vi "PictureCtrlDefault.vi"(1 "picture in":picture) -> (0 "Pause if TRUE":bool)   [LabVIEW 2020]
doc: "Displays the picture."
panel:
  out "Bad picture":T1
  out "picture out":picture
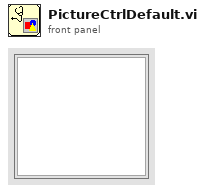
[diagram p1: front panel]
types:
  T1 = cluster{"Picture is empty or invalid":string, "Left:":i16, "Top:":i16, "Right:":i16, "Bottom:":i16}
  T2 = enum16{"Always On", "Always Off", "Off While Running"}
  T3 = typedef "imagedata.ctl" = cluster{"image type":i32, "image depth":i32, "image":u8[], "mask":u8[], "colors":u32[], "Rectangle":cluster{"left":i16, "top":i16, "right":i16, "bottom":i16}}
  T4 = typedef "LVBoundsTypeDef.ctl" = cluster{"Width":u32, "Height":u32}
  T5 = cluster{string, "left":i16, "top":i16, "right":i16, "bottom":i16}
  T6 = typedef "LVRectTypeDef.ctl" = cluster{"Left":i16, "Top":i16, "Right":i16, "Bottom":i16}
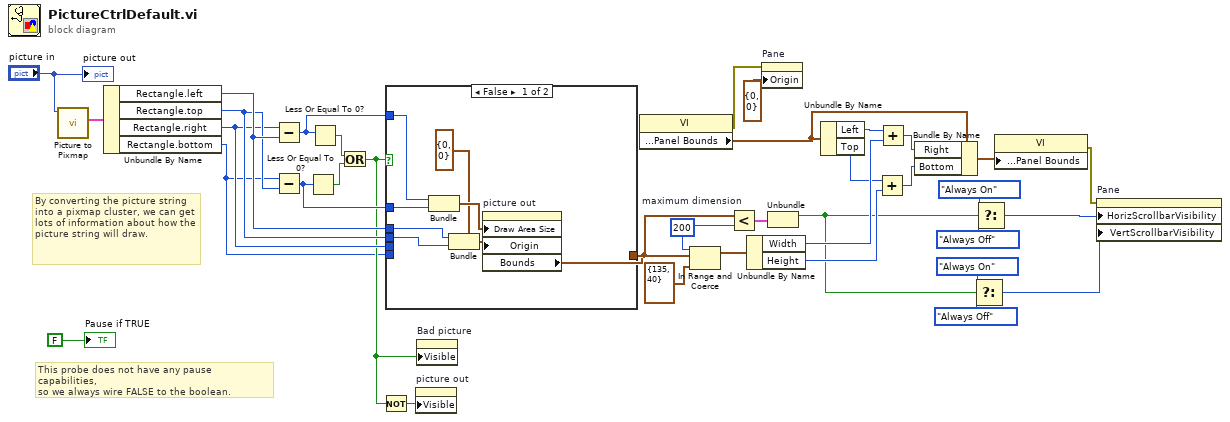
[diagram p0: block diagram]
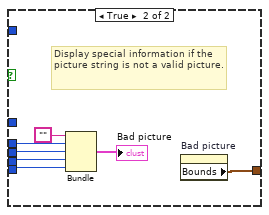
[diagram p2: hidden frame]
diagram:
  w17 = i16 200  # maximum dimension
  # "This probe does not have any pause capabilities,\nso we always wire FALSE to the boolean."
  # "By converting the picture string into a pixmap cluster, we can get lots of information about how the picture string will draw."
  n1 = call <vilib>:"Picture to Pixmap.vi"("picture"="picture in") -> ("image data"=w36:T3)  [unwired: 9 in, 1 out]
  n2 = Unbundle By Name(w36) -> ("Rectangle.left"=w32:i16, "Rectangle.top"=w31:i16, "Rectangle.right"=w30:i16, "Rectangle.bottom"=w13:i16)
  n3 = Subtract(x=w30, y=w32) -> (x-y=w29:i16)
  n4 = Subtract(x=w13, y=w31) -> (x-y=w28:i16)
  n5 = Less Or Equal To 0?(x=w28) -> (x <= 0?=w33:bool)
  n6 = Less Or Equal To 0?(x=w29) -> (x <= 0?=w34:bool)
  n7 = Or(x=w34, y=w33) -> (x .or. y?=w19:bool)
  n8 = Not(x=w19) -> (.not. x?=w18:bool)
  n9 = case shown="False" w19 {
    tunnel: w32 -> [w38 w50]
    tunnel: w31 -> [w37 w49]
    tunnel: w30 -> [_ w48]
    tunnel: w13 -> [_ w47]
    tunnel: [w41 w45] -> w16
    tunnel: w29 -> [w42 _]
    tunnel: w28 -> [w43 _]
    frame False {
      n10 = Bundle(w42, w43) -> (w44:cluster{i16, i16})  [unwired: 1 in]
      n11 = Bundle(cluster=cluster{"Horizontal":i16, "Vertical":i16} {"Horizontal"=0, "Vertical"=0} ("Origin"), "Horizontal"=w38, "Vertical"=w37) -> (w40:cluster{"Horizontal":i16, "Vertical":i16})
      n12 = property on="picture out" class="Pict"("Draw Area Size"=w44, "Origin"=w40) -> ("Bounds"=w41:T4)  [unwired: 2 in, 2 out]
    }
    frame True {
      # "Display special information if the picture string is not a valid picture."
      n13 = Bundle("", "left"=w50, "top"=w49, "right"=w48, "bottom"=w47) -> (→"Bad picture":T5)  [unwired: 1 in]
      n14 = property on="Bad picture" class="Clust (strict)"() -> ("Bounds"=w45:T4)  [unwired: 2 in, 2 out]
    }
  }
  n15 = property on="picture out" class="Pict"("Visible"=w18) -> ()  [unwired: 2 in, 2 out]
  n16 = property on="Bad picture" class="Clust (strict)"("Visible"=w19) -> ()  [unwired: 2 in, 2 out]
  n17 = property class="VI"() -> (error out=w12:errorcluster, "Front Panel Window:Panel Bounds"=w10:T6)  [unwired: 2 in, 1 out]
  n18 = In Range and Coerce(upper limit=w17, x=w16, lower limit=cluster{"Width":u32, "Height":u32} {"Width"=135, "Height"=40}) -> (coerced(x)=w21:T4)  [unwired: 1 out]
  n19 = Less?(x=w16, y=w17) -> (x < y?=w15:cluster{"Width":bool, "Height":bool})
  n20 = Unbundle By Name(w21) -> ("Width"=w26:u32, "Height"=w24:u32)
  n21 = property on="Pane" class="Pane"(error in=w12, "Origin"=cluster{"Horizontal":i16, "Vertical":i16} {"Horizontal"=0, "Vertical"=0} ("Front Panel Window:Origin")) -> ()  [unwired: 1 in, 2 out]
  n22 = Unbundle(w15) -> ("Width"=w1:bool)  [unwired: 1 out]
  n23 = Unbundle By Name(w10) -> ("Left"=w27:i16, "Top"=w25:i16)
  n24 = Add(x=w25, y=w24) -> (x+y=w9:u32)
  n25 = Add(x=w27, y=w26) -> (x+y=w23:u32)
  n26 = Bundle By Name(cluster=w10, "Right"=w23, "Bottom"=w9) -> (w22:T6)
  n27 = Select(t=T2."Always On" ("Horizontal Scrollbar Visibility"), s=w1, f=T2."Always Off" ("Horizontal Scrollbar Visibility")) -> (s? t:f=w2:T2)
  n28 = Select(t=T2."Always On" ("Horizontal Scrollbar Visibility"), s=w1, f=T2."Always Off" ("Horizontal Scrollbar Visibility")) -> (s? t:f=w6:T2)
  n29 = property class="VI"("Front Panel Window:Panel Bounds"=w22) -> (error out=w5:errorcluster)  [unwired: 2 in, 1 out]
  n30 = property on="Pane" class="Pane"(error in=w5, "HorizScrollbarVisibility"=w6, "VertScrollbarVisibility"=w2) -> ()  [unwired: 1 in, 2 out]
  "Pause if TRUE" <- FALSE ("Boolean")
  "picture out" <- "picture in"
